vi "AzCamParse.vi"(0 "InputString":string="OK arg1 arg2 arg3 arg4") -> (1 "Error":bool, 2 "Reply":string="arg4")   [LabVIEW 2014]
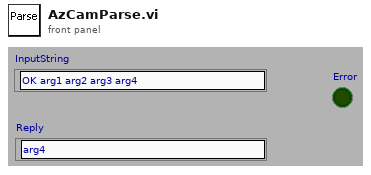
[diagram p1: front panel]
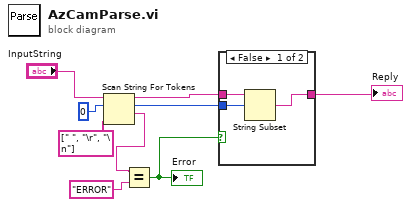
[diagram p0: block diagram]
diagram:
  n1 = Scan String For Tokens(6:string[] [" ", "\r", "\n"] ("delimiters (\\s,\\t,\\r,\\n)"), 8:0 ("offset"), 9:"InputString") -> (1:w5:string, 2:w4:i32, 3:w3:string)  [unwired: 3 in, 1 out]
  n2 = Equal?(x=w5, y="ERROR") -> (x = y?=w2:bool)
  "Error" <- w2
  n3 = case shown="False" w2 {
    tunnel: w4 -> [w12 _]
    tunnel: w3 -> [w11 w13]
    tunnel: [w10 w13] -> w1
    frame False {
      n4 = String Subset(string=w11, offset (0)=w12) -> (substring=w10:string)  [unwired: 1 in]
    }
    frame True {
    }
  }
  "Reply" <- w1
